vi "JSON RPC Engine.vi"(8 "error in (no error)":errorcluster) -> (0 "error out":errorcluster)   [LabVIEW 2016, in "JSONRPC Server.lvclass"]
doc: "Use this as a starting point for the RPC Server processing loop in your application"
uses:
  JSONRPC Server.lvclass
  Request/Request.lvclass/Request.ctl
  Request/request.Read method.vi
  Request/request.Read params.vi
  params/params.To JSON Tree.vi
  <vilib>/NI/JSON Support for LabVIEW/JSON Value/New JSON Value/New JSON (String).vi
  Add Response (Method Not Found from Request).vi
  Add Response (Result from Request).vi
  Add Response (Server Error from Request).vi
  Add Response (Internal Error from Request).vi
  <vilib>/NI/JSON Support for LabVIEW/JSON Value/JSON Value.lvclass
  Method Manager/Method Manager.lvclass
  Request/Request.lvclass
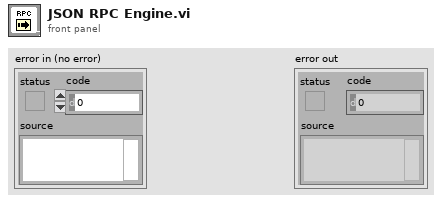
[diagram p1: front panel]
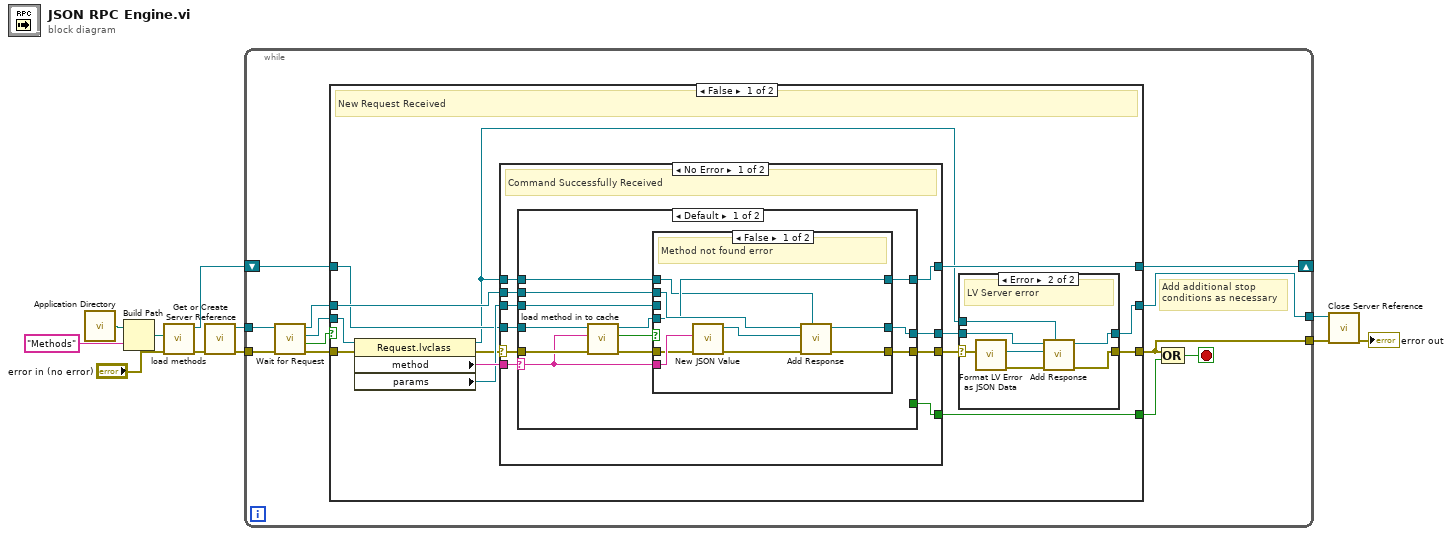
[diagram p0: block diagram]
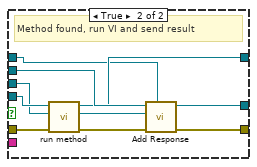
[diagram p3: hidden frame]
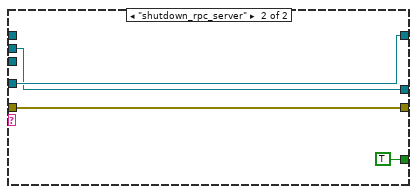
[diagram p4: hidden frame]
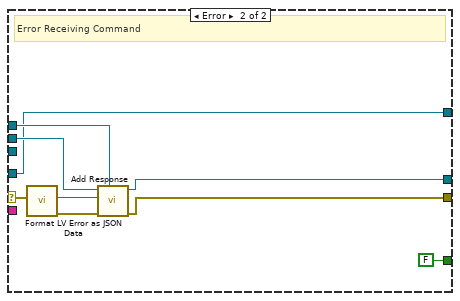
[diagram p5: hidden frame]
diagram:
  n1 = call <vilib>:"Application Directory.vi"() -> ("Application Directory"=w7:path)
  n2 = Build Path(base path=w7, name or relative path="Methods") -> (appended path=w5:path)
  n3 = call "load methods.vi"("error in (no error)"="error in (no error)", "Folder Path"=w5) -> ("error out"=w4:errorcluster, "Method Manager out"=w3:refnum<class "Method Manager.lvclass">)  [unwired: 8 in]
  n4 = call "Get or Create Server Reference.vi"("error in (no error)"=w4) -> ("error out"=w10:errorcluster, "Server Out"=w11:refnum<class "JSONRPC Server.lvclass">)  [unwired: 9 in]
  n5 = while {
    tunnel: w11 -> [w23]
    tunnel: w10 -> [w19]
    tunnel: [w15] -> w8
    tunnel: [w17] -> w9
    shift-right: [w12] -> _
    shift-left: w3 -> [w13]
    stop <- w14 stop-if-true
    # "Add additional stop\nconditions as necessary"
    n6 = call "Wait for Request.vi"("error in (no error)"=w19, "Server in"=w23) -> ("error out"=w18:errorcluster, "timed out?"=w20:bool, "Request"=w21:refnum<class "Request.lvclass">, "Server out"=w22:refnum<class "JSONRPC Server.lvclass">)  [unwired: 6 in]
    n7 = case shown="False" w20 {
      tunnel: w22 -> [w31 w102]
      tunnel: w21 -> [w37 _]
      tunnel: w18 -> [w34 w103]
      tunnel: [w27 w103] -> w15
      tunnel: [w32 _] -> w16
      tunnel: [w25 w102] -> w17
      tunnel: w13 -> [w30 w101]
      tunnel: [w29 w101] -> w12
      frame False {
        # "New Request Received"
        n8 = property class="Request.lvclass"(reference=w37, error in=w34) -> (reference out=w24:refnum<class "Request.lvclass">, error out=w33:errorcluster, "method"=w36:string, "params"=w35:refnum<class "JSON Value.lvclass">)
        n9 = case shown="No Error" w33 {
          selector: w33 -> [w54 w94]
          tunnel: w36 -> [w56 _]
          tunnel: w35 -> [w47 _]
          tunnel: [w51 w97] -> w28
          tunnel: [w50 FALSE] -> w32
          tunnel: w31 -> [w53 w99]
          tunnel: [w49 w98] -> w26
          tunnel: w24 -> [w48 w100]
          tunnel: w30 -> [w55 w92]
          tunnel: [w52 w92] -> w29
          frame No Error {
            # "Command Successfully Received"
            n10 = case shown="Default" w56 {
              selector: w56 -> [w58 _]
              tunnel: w55 -> [w68 w91]
              tunnel: w54 -> [w64 w90]
              tunnel: w53 -> [w63 w88]
              tunnel: [w62 w91] -> w52
              tunnel: [w60 w90] -> w51
              tunnel: [_ TRUE] -> w50
              tunnel: [w61 w88] -> w49
              tunnel: w48 -> [w59 _]
              tunnel: w47 -> [w57 _]
              frame Default {
                n11 = call "load method in to cache.vi"("error in (no error)"=w64, "method name"=w58, "Method Manager in"=w68) -> ("error out"=w65:errorcluster, "found?"=w67:bool, "Method Manager out"=w66:refnum<class "Method Manager.lvclass">)  [unwired: 6 in]
                n12 = case shown="False" w67 {
                  tunnel: w66 -> [w70 w87]
                  tunnel: w65 -> [w76 w86]
                  tunnel: w63 -> [w74 w85]
                  tunnel: [w70 w82] -> w62
                  tunnel: [w73 w80] -> w61
                  tunnel: [w71 w81] -> w60
                  tunnel: w59 -> [w69 w79]
                  tunnel: w58 -> [w77 _]
                  tunnel: w57 -> [_ w78]
                  frame False {
                    # "Method not found error"
                    n13 = call-poly <vilib>:"New JSON Value.vi"("error in (no error)"=w76, "value"=w77) -> ("error out"=w72:errorcluster, "JSON Value out"=w75:refnum<class "JSON Value.lvclass">)  [unwired: 8 in]
                    n14 = call-poly "Add Response.vi"("Request"=w69, "error in (no error)"=w72, "data"=w75, "Server in"=w74) -> ("error out"=w71:errorcluster, "Server out"=w73:refnum<class "JSONRPC Server.lvclass">)  [unwired: 5 in, 1 out]
                  }
                  frame True {
                    # "Method found, run VI and send result"
                    n15 = call "run method.vi"("error in (no error)"=w86, "JSON Value in"=w78, "Method Manager in"=w87) -> ("error out"=w84:errorcluster, "JSON Value out"=w83:refnum<class "JSON Value.lvclass">, "Method Manager out"=w82:refnum<class "Method Manager.lvclass">)  [unwired: 6 in]
                    n16 = call-poly "Add Response.vi"("Request"=w79, "error in (no error)"=w84, "JSON Value in"=w83, "Server in"=w85) -> ("error out"=w81:errorcluster, "Server out"=w80:refnum<class "JSONRPC Server.lvclass">)  [unwired: 5 in, 1 out]
                  }
                }
              }
              frame "shutdown_rpc_server" {
              }
            }
          }
          frame Error {
            # "Error Receiving Command"
            n17 = call "Format LV Error as JSON Data.vi"("error in"=w94) -> ("error out"=w95:errorcluster, "Error Value out"=w93:refnum<class "JSON Value.lvclass">)  [unwired: 9 in]
            n18 = call-poly "Add Response.vi"("Request"=w100, "error in (no error)"=w95, "data"=w93, "Server in"=w99) -> ("error out"=w97:errorcluster, "Server out"=w98:refnum<class "JSONRPC Server.lvclass">)  [unwired: 5 in, 1 out]
          }
        }
        n19 = case shown="Error" w28 {
          selector: w28 -> [w39 w42]
          tunnel: [w39 w41] -> w27
          tunnel: w26 -> [w38 w45]
          tunnel: [w38 w44] -> w25
          tunnel: w24 -> [_ w40]
          frame No Error {
          }
          frame Error {
            # "LV Server error"
            n20 = call "Format LV Error as JSON Data.vi"("error in"=w42) -> ("error out"=w43:errorcluster, "Error Value out"=w46:refnum<class "JSON Value.lvclass">)  [unwired: 9 in]
            n21 = call-poly "Add Response.vi"("Request"=w40, "error in (no error)"=w43, "data"=w46, "Server in"=w45) -> ("error out"=w41:errorcluster, "Server out"=w44:refnum<class "JSONRPC Server.lvclass">)  [unwired: 5 in, 1 out]
          }
        }
      }
      frame True {
        # "Timeout while waiting for new Requests"
      }
    }
    n22 = Compound Arithmetic op=OR(w15, w16) -> (w14:bool)
  }
  n23 = call "Close Server Reference.vi"("error in (no error)"=w8, "Server in"=w9) -> ("error out"=→"error out":errorcluster)  [unwired: 9 in]
